vi "Stop.vi"(8 "error in (no error)":errorcluster) -> (0 "error out":errorcluster)   [LabVIEW 2017, in "MCSA_9065_API.lvlib"]
uses:
  <vilib>/addons/InsightCM/Devices/Shared/Mcsa/Fpga/McsaAcquire/subVIs/McsaAPI_9065/MCSA_9065_API.lvlib
  <vilib>/eio/EIONode/EIONode.xnode
  <vilib>/rvi/eio/common/nirviEmuTemplateMethod_errors.vi
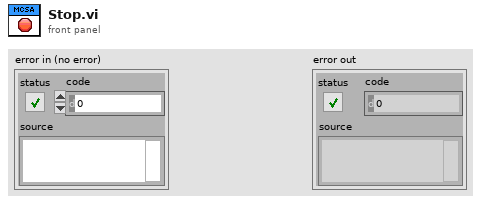
[diagram p1: front panel]
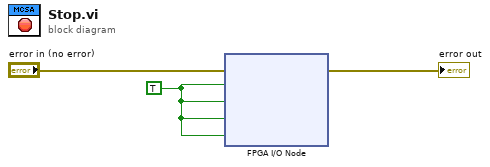
[diagram p0: block diagram]
diagram:
  w1 = TRUE ("Mod1/Start")
  n1 = xnode "FPGA I/O Node"("error in"="error in (no error)", "Mod1/Stop"=w1, "Mod2/Stop"=w1, "Mod3/Stop"=w1, "Mod4/Stop"=w1) -> ("error out"=→"error out":errorcluster)  [unwired: 4 in, 4 out]
